vi "LbcbFactory.vi"(8 "error in (no error)":errorcluster, 9 "LbcbConversionType":T1, 10 "LBCB Number":T2, 11 "Actions":T3) -> (0 "error out":errorcluster)   [LabVIEW 2013]
uses:
  W:/Operations Manager New DLL/DLL/LbcbConversions.dll
  DLL/LbcbConversions.dll
  Data Access Objects/Metadata/Persistant DAO Actions.ctl
  Data Access Objects/Metadata/LBCB Number.ctl
  Data Access Objects/Metadata/DAO Actions with Remove.ctl
  LbcbConversionTypes.ctl
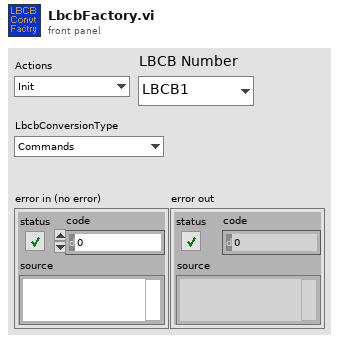
[diagram p1: front panel]
types:
  T1 = typedef "LbcbConversionTypes.ctl" = enum16{"Commands", "Readings", "Offsets"}
  T2 = typedef "LBCB Number.ctl" = enum16{"LBCB1", "LBCB2"}
  T3 = typedef "DAO Actions with Remove.ctl" = enum16{"Init", "Get", "Set", "Remove"}
  T4 = typedef "Persistant DAO Actions.ctl" = enum16{"Init", "Get", "Set", "Load", "Save"}
  T5 = typedef "LBCB Position.ctl" = cluster{"Motion Center":dbl[], "Transformation Matrix":dbl[][]}
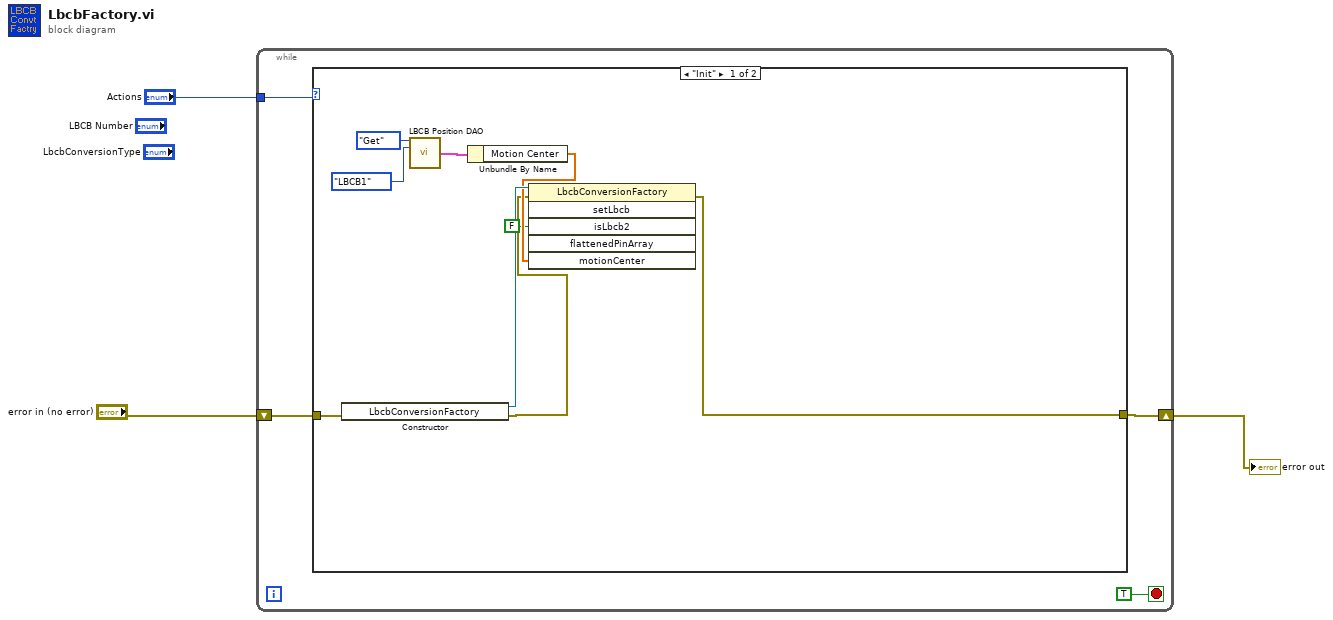
[diagram p0: block diagram]
diagram:
  n1 = while {
    tunnel: "Actions" -> [w6]
    shift-right: [w4] -> w1
    shift-left: "error in (no error)" -> [w5]
    stop <- TRUE stop-if-true
    n2 = case shown="\"Init\"" w6 {
      tunnel: w5 -> [w16 _]
      tunnel: [w10 _] -> w4
      frame "Init" {
        n3 = constructor class="LbcbConversionFactory"(error in=w16) -> (reference out=w15:refnum<k24>, error out=w11:errorcluster)  [unwired: 2 in, 1 out]
        n4 = call "LBCB Position DAO.vi"("LBCB Settings Actions"=Persistant_DAO_Actions."Get", "LBCB Number"=LBCB_Number."LBCB1") -> ("LBCB Position Output"=w13:T5)  [unwired: 11 in, 2 out]
        n5 = Unbundle By Name(w13) -> ("Motion Center"=w12:dbl[])
        n6 = invoke class="LbcbConversionFactory" method="setLbcb"(reference=w15, error in=w11, "isLbcb2"=FALSE, "motionCenter"=w12) -> (error out=w10:errorcluster)  [unwired: 2 in, 5 out]
      }
      frame "Get" {
      }
    }
  }
  "error out" <- w1
